vi "Get Num Axes.vi"(8 "error in (no error)":errorcluster) -> (0 "error out":errorcluster, 3 "num-axes":i32)   [LabVIEW 2020, in "Manipulator CLI Driver.lvlib"]
uses:
  Manipulator CLI Driver.lvlib
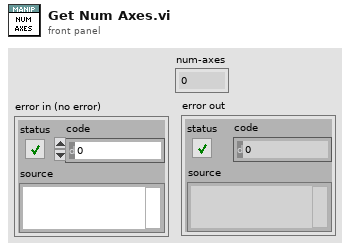
[diagram p1: front panel]
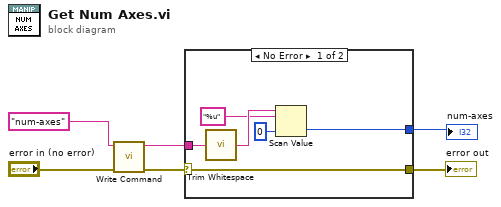
[diagram p0: block diagram]
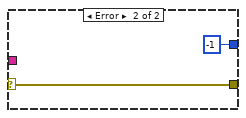
[diagram p2: hidden frame]
diagram:
  n1 = call "Write Command.vi"("error in (no error)"="error in (no error)", "command"="num-axes") -> ("error out"=w4:errorcluster, "standard output"=w2:string)  [unwired: 7 in, 1 out]
  n2 = case shown="No Error" w4 {
    selector: w4 -> [w12 w14]
    tunnel: [w12 w14] -> w3
    tunnel: w2 -> [w11 _]
    tunnel: [w8 -1 ("default (0 dbl)")] -> w1
    frame No Error {
      n3 = call <vilib>:"Trim Whitespace.vi"("string"=w11) -> ("trimmed string"=w10:string)  [unwired: 1 in]
      n4 = Scan Value(string=w10, format string="%u", default (0 dbl)=0) -> (value=w8:i32)  [unwired: 1 out]
    }
    frame Error {
    }
  }
  "error out" <- w3
  "num-axes" <- w1
